vi "ge_Read Lines From File.vi"(0 "file path (dialog if empty)":path, 2 "convert eol? (no:F)":bool, 5 "number of lines (all:-1)":i32=-1, 7 "start of read offset (chars.:0)":i32, 9 "[max characters per line]  (no limit:0)":i32, 11 "error in":errorcluster) -> (4 "new file path (Not A Path if cancelled)":path, 6 "line string":string, 8 "mark after read (chars.)":i32, 10 "EOF?":bool, 15 "error out":errorcluster)   [LabVIEW 2018]
doc: "LabVIEW no longer supports this VI. Use the Read Text function instead. Reads a specified number of lines from a byte stream file beginning at a specified character offset. The VI opens the file before reading from it and closes it afterwards."
panel:
  in  "prompt":string="Choose file to read."
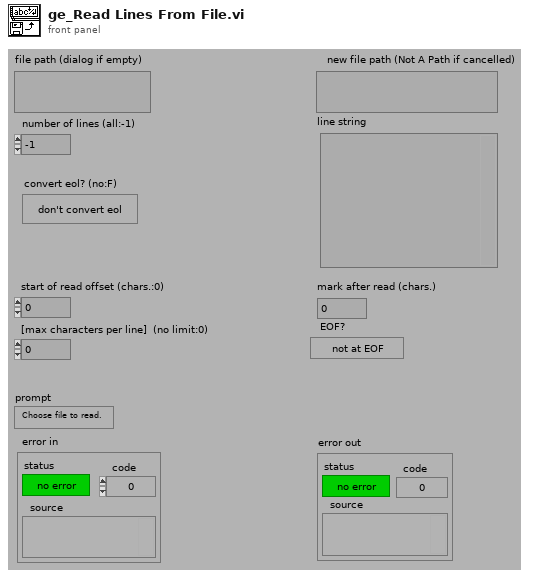
[diagram p1: front panel]
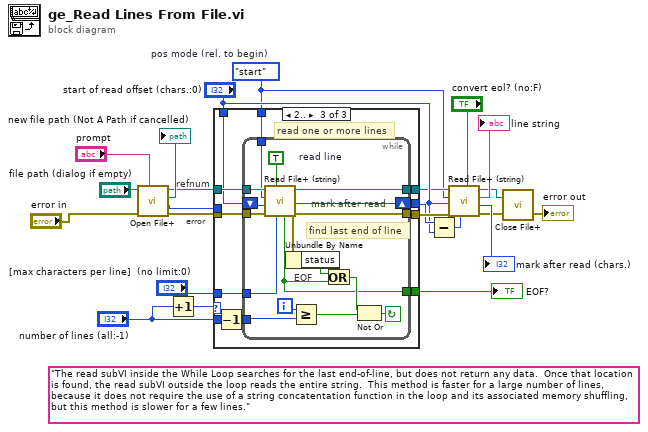
[diagram p0: block diagram]
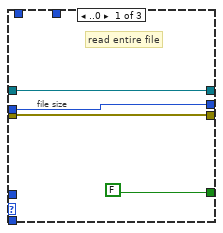
[diagram p2: hidden frame]
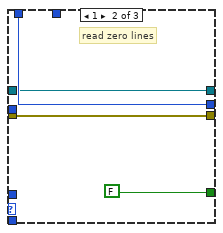
[diagram p3: hidden frame]
diagram:
  w11 = enum16{"start", "end", "current"}."start"  # pos mode (rel. to begin)
  (unwired) "The read subVI inside the While Loop searches for the last end-of-line, but does not return any data.  Once that location is found, the read subVI outside the loop reads the entire string.  This method is faster for a large number of lines, because it does not require the use of a string concatentation function in the loop and its associated memory shuffling, but this method is slower for a few lines."
  # "error"
  # "refnum"
  n1 = call <vilib>:"Open File+.vi"("prompt"="prompt", "error in (not an error)"="error in", "file path (\" \")"="file path (dialog if empty)") -> ("error out"=w10:errorcluster, "file size (bytes)"=w9:i32, "file path"=→"new file path (Not A Path if cancelled)":path, "refnum"=w7:refnum<file>)  [unwired: 5 in]
  n2 = Increment(x="number of lines (all:-1)") -> (x+1=w17:i32)
  n3 = case shown="2.." w17 {
    tunnel: [w27 w30 w42] -> w19
    tunnel: [w26 w31 w41] -> w18
    tunnel: "number of lines (all:-1)" -> [_ _ w40]
    tunnel: "[max characters per line]  (no limit:0)" -> [_ _ w39]
    tunnel: w10 -> [w27 w30 w38]
    tunnel: w7 -> [w25 w29 w37]
    tunnel: "start of read offset (chars.:0)" -> [_ w31 w36]
    tunnel: w11 -> [_ _ w35]
    tunnel: w9 -> [w26 _ _]
    tunnel: [w25 w29 w34] -> w14
    tunnel: [FALSE FALSE w33] -> w13
    frame ..0 {
      # "file size"
      # "read entire file"
    }
    frame 1 {
      # "read zero lines"
    }
    frame 2.. {
      # "read one or more lines"
      n4 = Decrement(x=w40) -> (x-1=w32:i32)
      n5 = while {
        tunnel: [w44] -> w33
        tunnel: w35 -> [w49]
        tunnel: w38 -> [w51]
        tunnel: w39 -> [w52]
        tunnel: [w47] -> w42
        tunnel: w37 -> [w54]
        tunnel: [w55] -> w34
        tunnel: w32 -> [w43]
        shift-left: w36 -> [w56]
        shift-right: [w58] -> w41
        i -> [w57]
        stop <- w50 continue-if-true
        w46 = TRUE  # read line
        # "mark after read"
        # "find last end of line"
        # "EOF"
        n6 = call <vilib>:"Read File+ (string).vi"("count"=w52, "line mode (characters:F)"=w46, "error in (no error)"=w51, "pos offset (bytes:0)"=w56, "pos mode (rel. to current:2)"=w49, "refnum"=w54) -> ("error out"=w47:errorcluster, "mark after read (bytes)"=w58:i32, "dup refnum"=w55:refnum<file>, "EOF?"=w44:bool)  [unwired: 1 in, 1 out]
        n7 = Unbundle By Name(w47) -> ("status"=w45:bool)
        n8 = Greater Or Equal?(x=w57, y=w43) -> (x >= y?=w53:bool)
        n9 = Or(x=w45, y=w44) -> (x .or. y?=w48:bool)
        n10 = Not Or(1:w53, 2:w48) -> (0:w50:bool)
      }
    }
  }
  "EOF?" <- w13
  n11 = Subtract(x=w18, y="start of read offset (chars.:0)") -> (x-y=w23:i32)
  n12 = call <vilib>:"Read File+ (string).vi"("convert eol? (no:F)"="convert eol? (no:F)", "count"=w23, "error in (no error)"=w19, "pos offset (bytes:0)"="start of read offset (chars.:0)", "pos mode (rel. to current:2)"=w11, "refnum"=w14) -> ("error out"=w4:errorcluster, "mark after read (bytes)"=→"mark after read (chars.)":i32, "string"=→"line string":string, "dup refnum"=w3:refnum<file>)  [unwired: 1 in, 1 out]
  n13 = call <vilib>:"Close File+.vi"("error in (no error)"=w4, "refnum"=w3) -> ("error out"=→"error out":errorcluster)  [unwired: 3 in, 2 out]
